vi "Pre Launch Init.vi"(11 "Machine d'état in":refnum<class "Machine d'état.lvclass">) -> (0 "error out":errorcluster, 3 "Machine d'état out":refnum<class "Machine d'état.lvclass">)   [LabVIEW 2020, in "Machine d'état.lvlib" / "Machine d'état.lvclass"]
doc: "(<B>Filename</B>: Actor Framework.lvlib:Actor.lvclass:Pre Launch Init.vi)\n\nDefines behavior that occurs after the Launch Nested Actor method is invoked but before the actor's Actor Core method begins running.\n\nBy default, this method does nothing. A descendant class may override it to define behavior."
uses:
  <vilib>/ActorFramework/Actor/Actor.lvclass
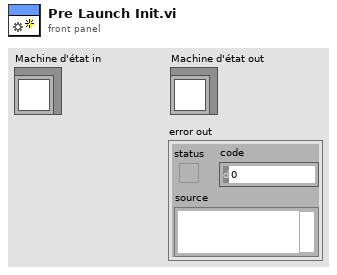
[diagram p1: front panel]
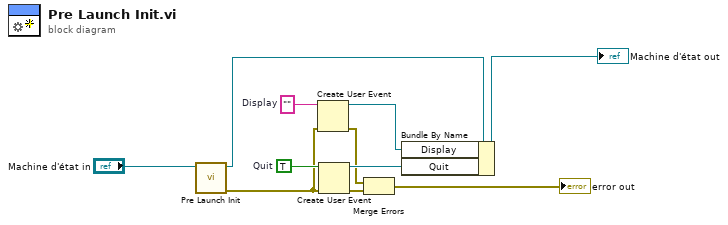
[diagram p0: block diagram]
diagram:
  w2 = ""  # Display
  w9 = TRUE  # Quit
  n1 = call-parent "Pre Launch Init.vi"("Actor in"="Machine d'état in") -> ("error out"=w5:errorcluster, "Actor out"=w11:refnum<class "Machine d'état.lvclass">)  [unwired: 9 in]
  n2 = Create User Event(user event datatype=w2, error in=w5) -> (user event=w1:refnum<user-event>, error out=w3:errorcluster)
  n3 = Create User Event(user event datatype=w9, error in=w5) -> (user event=w7:refnum<user-event>, error out=w6:errorcluster)
  n4 = Merge Errors(w3, w6) -> (→"error out":errorcluster)
  n5 = Bundle By Name(cluster=w11, "Display"=w1, "Quit"=w7) -> (→"Machine d'état out":refnum<class "Machine d'état.lvclass">)
